vi "Halton Sequence.vi"(7 "initialize?":bool=TRUE, 10 "seed":i32=3, 11 "samples":i32=128) -> (0 "error":i32, 3 "Halton Pattern":dbl[](array[numeric]))   [LabVIEW 2017, in "NI_AAL_SignalGeneration.lvlib"]
doc: "Generates quasi-random Halton or Richtmeyer sequences, which are low-discrepancy number sequences."
uses:
  <vilib>/Analysis/NI_AAL_SignalGeneration.lvlib
  <vilib>/gmath/NI_AAL_MathFunc.lvlib
panel:
  # "Halton Sequence"
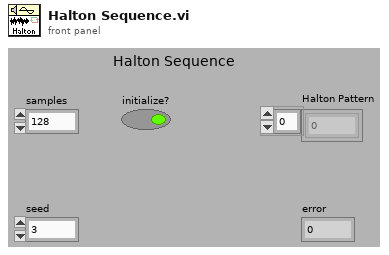
[diagram p1: front panel]
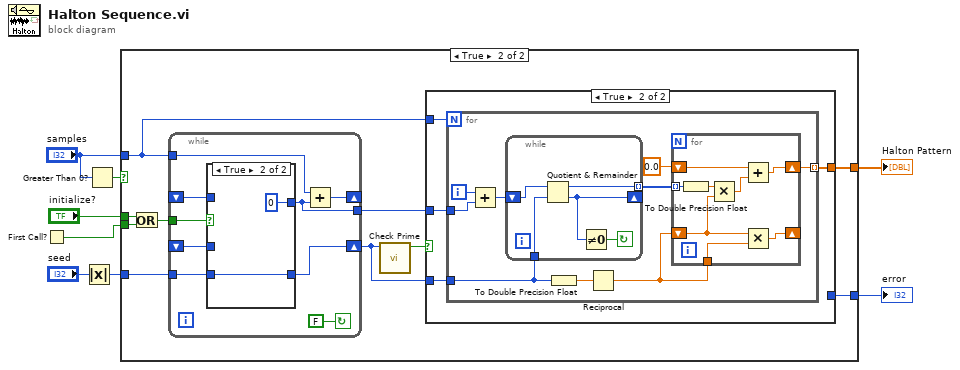
[diagram p0: block diagram]
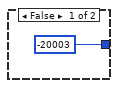
[diagram p2: hidden frame]
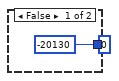
[diagram p3: hidden frame]
diagram:
  n1 = First Call?() -> (First Call?: T/F=w6:bool)
  n2 = Absolute Value(x="seed") -> (abs(x)=w2:i32)
  n3 = Greater Than 0?(x="samples") -> (x > 0?=w4:bool)
  n4 = case shown="True" w4 {
    tunnel: w2 -> [_ w19]
    tunnel: [_ w18] -> w8
    tunnel: [-20003 w10] -> w1
    tunnel: "samples" -> [_ w16]
    tunnel: "initialize?" -> [_ w15]
    tunnel: w6 -> [_ w14]
    frame False {
    }
    frame True {
      n5 = Or(x=w15, y=w14) -> (x .or. y?=w13:bool)
      n6 = while {
        shift-right: [w53] -> _
        shift-left: _ -> [w55]
        tunnel: w19 -> [w49]
        shift-right: [w50] -> w17
        shift-left: _ -> [w51]
        tunnel: w16 -> [w52]
        tunnel: [w48] -> w11
        tunnel: w13 -> [w47]
        stop <- FALSE continue-if-true
        n7 = case shown="True" w47 {
          tunnel: w55 -> [w57 _]
          tunnel: [w57 0] -> w48
          tunnel: w51 -> [w56 _]
          tunnel: [w56 w58] -> w50
          tunnel: w49 -> [_ w58]
          frame False {
          }
          frame True {
          }
        }
        n8 = Add(x=w52, y=w48) -> (x+y=w53:i32)
      }
      n9 = call <vilib>:"Check Prime.vi"("n"=w17) -> ("prime?"=w12:bool)  [unwired: 10 in]
      n10 = case shown="True" w12 {
        tunnel: w16 -> [_ w23]
        tunnel: w17 -> [_ w24]
        tunnel: [_ w22] -> w18
        tunnel: w11 -> [_ w21]
        tunnel: [-20130 _] -> w10
        frame False {
          (unwired) 0
          (unwired) -20061
        }
        frame True {
          n11 = for {
            N: w23 -> [_]
            tunnel: w24 -> [w30]
            tunnel: [w29] -> w22 mode=indexing
            tunnel: w21 -> [w26]
            i -> [w27]
            n12 = Add(x=w27, y=w26) -> (x+y=w28:i32)
            n13 = while {
              tunnel: [w37] -> w33 mode=indexing
              tunnel: w30 -> [w38]
              shift-left: w28 -> [w36]
              shift-right: [w35] -> _
              stop <- w34 continue-if-true
              n14 = Quotient & Remainder(x=w36, y=w38) -> (x-y*floor(x/y)=w37:i32, floor(x/y)=w35:i32)
              n15 = Not Equal To 0?(x=w35) -> (x != 0?=w34:bool)
            }
            n16 = To Double Precision Float(number=w30) -> (double precision float=w25:dbl)
            n17 = Reciprocal(x=w25) -> (1/x=w32:dbl)
            n18 = for {
              shift-right: [w40] -> w29
              shift-left: 0.0 -> [w42]
              shift-right: [w45] -> _
              shift-left: w32 -> [w44]
              tunnel: w32 -> [w46]
              tunnel: w33 -> [w43] mode=indexing
              n19 = To Double Precision Float(number=w43) -> (double precision float=w39:dbl)
              n20 = Multiply(x=w39, y=w44) -> (x*y=w41:dbl)
              n21 = Add(x=w42, y=w41) -> (x+y=w40:dbl)
              n22 = Multiply(x=w44, y=w46) -> (x*y=w45:dbl)
            }
          }
        }
      }
    }
  }
  "Halton Pattern" <- w8
  "error" <- w1
